vi "Continuous Input and Output.vi"() -> ()   [LabVIEW 2014]
doc: "This example demonstrates how to continuously acquire buffered voltage measurements using a DAQmx device.\n\nFor instructions on how to connect your signals to the DAQ device, refer to your device documentation."
uses:
  <vilib>/Utility/error.llb/DialogType.ctl
  <vilib>/DAQmx/read.llb/DAQmx Read (Analog 1D Wfm NChan NSamp).vi
  <vilib>/DAQmx/write.llb/DAQmx Write (Analog 1D DBL NChan 1Samp).vi
  <vilib>/DAQmx/create/channels.llb/DAQmx Create Channel (AI-Voltage-Basic).vi
  <vilib>/DAQmx/configure/timing.llb/DAQmx Timing (Sample Clock).vi
  <vilib>/DAQmx/create/channels.llb/DAQmx Create Channel (AO-Voltage-Basic).vi
  <vilib>/DAQmx/miscellaneous.llb/DAQmx Fill In Error Info.vi
  <vilib>/measure/madcrms.llb/Basic Averaged DC-RMS for 1 Chan.vi
  <vilib>/express/express analysis/Spectral/Block/exnSpectralBlock spectral measurements power poly.vi
  <vilib>/express/express analysis/Spectral/Block/exnSpectralBlock spectral measurements power WFM.vi
  <vilib>/express/express analysis/Spectral/XNode/ExpressSpectralMeasurementsBlockNode.xnode
  <resource>/objmgr/daqmx.rc
  <vilib>/measure/NI_MAPro.lvlib
panel:
  in  "Lower Cut-Off":dbl=100.0
  in  "Channel to Filter":i32
  out "Spectrum":cluster{"f0":dbl, "df":dbl, "magnitude":dbl[]}(graph)
  out "Filtered Data":waveform(dbl)(graph)
  in  "Physical Channel(s)":tag="Dev1/ao0"
  in  "Stop":bool
  out "Waveform Graph":waveform(dbl)[](graph)
  in  "Number of Samples":i32=100
  in  "Sample Rate":dbl=1000.0
  in  "Sample Clock Source":tag="OnboardClock"
  in  "Terminal Configuration":i32(ring)=-1 items=["default"=-1, "RSE"=10083, "NRSE"=10078, "Differential"=10106, "Pseudodifferential"=12529]
  in  "Max Voltage":dbl=5.0
  in  "Min Voltage":dbl
  in  "Physical Input Channel":tag="Dev1/ai0"
  out "Actual Sample Rate":dbl=1000.0 format="%0.2f"
  # "Channel Settings"
  # "Acquired Data"
  # "Filtered Data"
  # "Timing Settings"
  # "Spectrum"
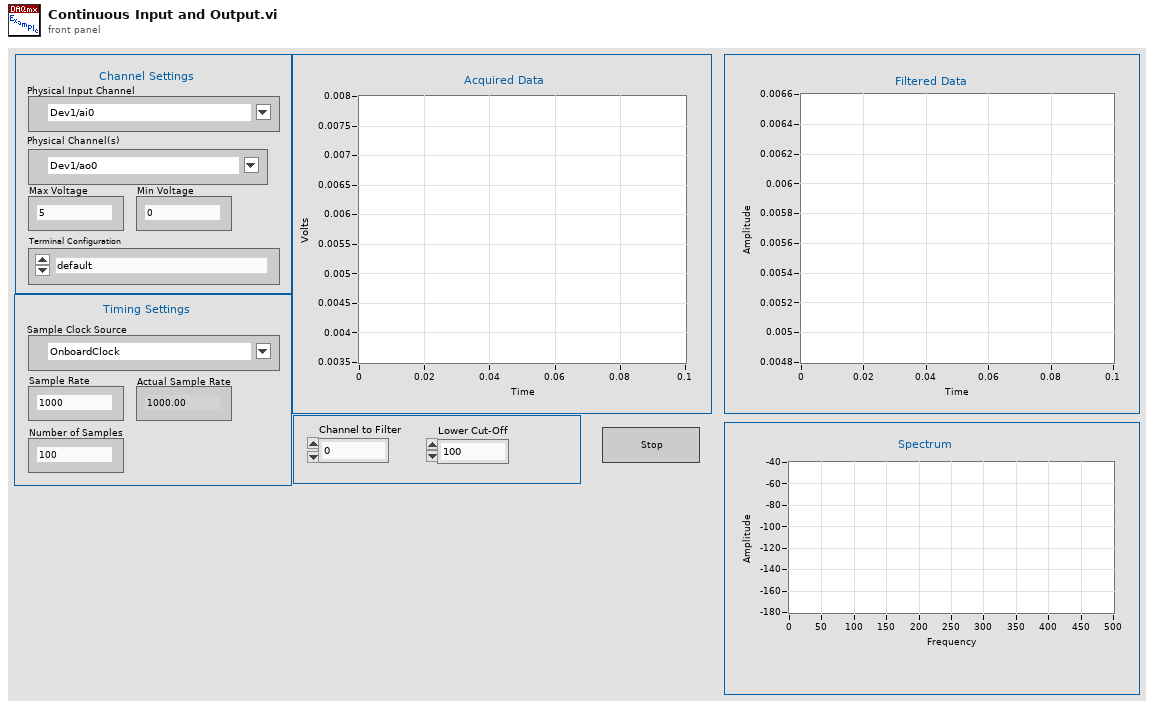
[diagram p1: front panel]
types:
  T1 = typedef "DialogType.ctl" = u16
  T2 = cluster{"averaging mode":u16, "weighting mode":u16, "number of averages":u32}
  T3 = cluster{"dB On (F)":bool, "unwrap phase (F)":bool, "convert to degree (F)":bool}
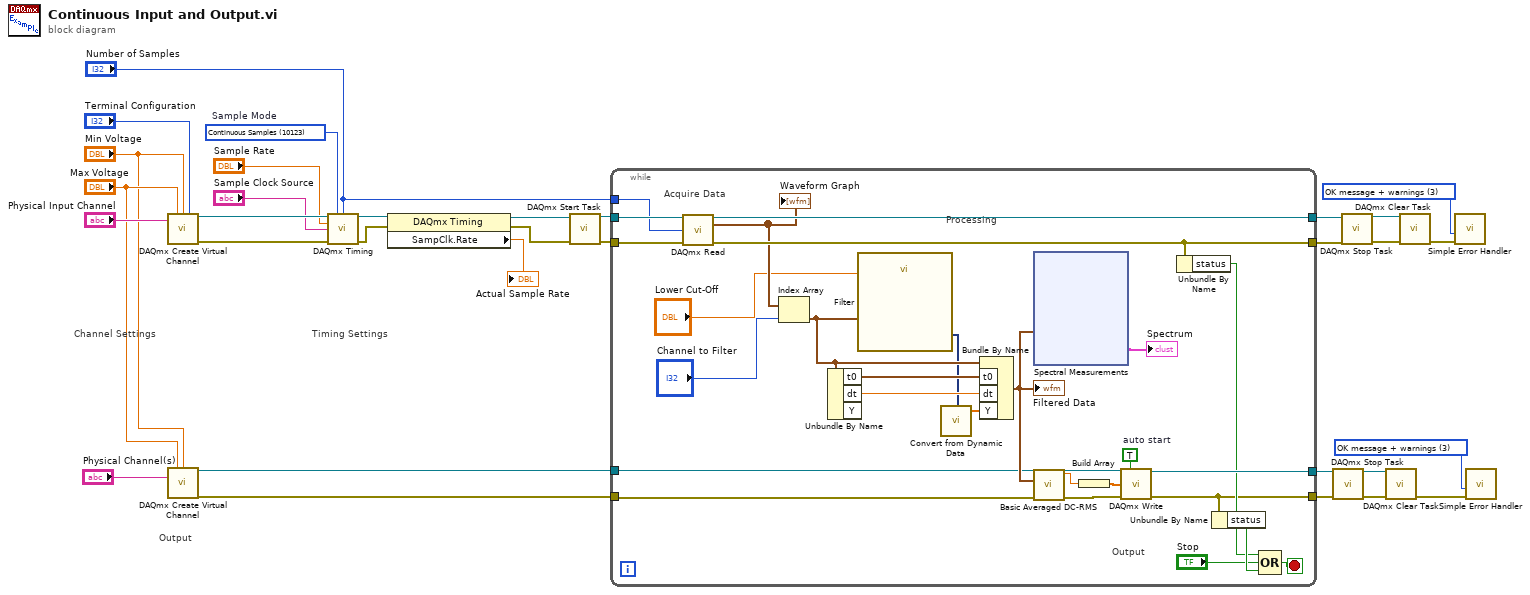
[diagram p0: block diagram]
diagram:
  w7 = T1 3 items=["no dialog", "OK message", "continue or stop message", "OK message + warnings", "continue/stop + warnings"] ("type of dialog (OK msg:1)")
  w17 = T1 3 items=["no dialog", "OK message", "continue or stop message", "OK message + warnings", "continue/stop + warnings"] ("type of dialog (OK msg:1)")
  w11 = 10123 items=["Finite Samples"=10178, "Continuous Samples"=10123, "Hardware Timed Single Point"=12522]  # Sample Mode
  # "Output"
  # "Timing Settings"
  # "Channel Settings"
  n1 = call-poly <vilib>:"DAQmx Create Virtual Channel.vi"("maximum value"="Max Voltage", "minimum value"="Min Voltage", "input terminal configuration"="Terminal Configuration", "physical channels"="Physical Input Channel") -> ("task out"=w29:refnum<k21>, "error out"=w30:errorcluster)  [unwired: 10 in]
  n2 = call-poly <vilib>:"DAQmx Create Virtual Channel.vi"("maximum value"="Max Voltage", "minimum value"="Min Voltage", "physical channels"="Physical Channel(s)") -> ("task out"=w2:refnum<k21>, "error out"=w1:errorcluster)  [unwired: 11 in]
  n3 = call-poly <vilib>:"DAQmx Timing.vi"("task/channels in"=w29, "sample mode"=w11, "samples per channel"="Number of Samples", "rate"="Sample Rate", "source"="Sample Clock Source", "error in"=w30) -> ("task out"=w32:refnum<k21>, "error out"=w31:errorcluster)  [unwired: 8 in]
  n4 = property class="DAQmx Timing"(reference=w32, error in=w31) -> (reference out=w4:refnum<k21>, error out=w3:errorcluster, "SampClk.Rate"=→"Actual Sample Rate":dbl)
  n5 = call <vilib>:"DAQmx Start Task.vi"("task/channels in"=w4, "error in"=w3) -> ("task out"=w28:refnum<k21>, "error out"=w27:errorcluster)  [unwired: 12 in]
  n6 = while {
    tunnel: w28 -> [w59]
    tunnel: w27 -> [w58]
    tunnel: [w57] -> w21
    tunnel: [w56] -> w20
    tunnel: "Number of Samples" -> [w55]
    tunnel: [w54] -> w6
    tunnel: [w39] -> w5
    tunnel: w2 -> [w34]
    tunnel: w1 -> [w33]
    stop <- w50 stop-if-true
    w38 = TRUE  # auto start
    # "Output"
    # "Processing"
    # "Acquire Data"
    n7 = call-poly <vilib>:"DAQmx Read.vi"("task/channels in"=w59, "number of samples per channel"=w55, "error in"=w58) -> ("task out"=w57:refnum<k21>, "data"=w49:waveform(dbl)[], "error out"=w56:errorcluster)  [unwired: 10 in]
    "Waveform Graph" <- w49
    n8 = Index Array(array=w49, index="Channel to Filter") -> (element=w47:waveform(dbl))
    n9 = Unbundle By Name(w47) -> ("t0"=w46:timestamp, "dt"=w45:dbl)  [unwired: 1 out]
    n10 = call "Filter"("Lower Cut-Off"="Lower Cut-Off", "Signal"=w47) -> ("Filtered Signal"=w40:dynamicdata)  [unwired: 8 in, 1 out]
    n11 = call "Convert from Dynamic Data"("Dynamic Data Type"=w40) -> ("Array"=w44:dbl[])  [unwired: 3 in]
    n12 = Bundle By Name(cluster=w47, "t0"=w46, "dt"=w45, "Y"=w44) -> (w42:waveform(dbl))
    "Filtered Data" <- w42
    n13 = xnode "Spectral Measurements"("Signals"=w42) -> ("Power Spectrum"=→"Spectrum":cluster{"f0":dbl, "df":dbl, "magnitude":dbl[]})  [unwired: 1 in, 1 out]
    n14 = call-poly <vilib>:"Basic Averaged DC-RMS.vi"("error in (no error)"=w33, "signal in"=w42) -> ("error out"=w37:errorcluster, "DC value"=w36:dbl)  [unwired: 6 in, 2 out]
    n15 = Build Array(w36) -> (w35:dbl[])
    n16 = call-poly <vilib>:"DAQmx Write.vi"("task/channels in"=w34, "auto start"=w38, "data"=w35, "error in"=w37) -> ("task out"=w54:refnum<k21>, "error out"=w39:errorcluster)  [unwired: 9 in, 1 out]
    n17 = Unbundle By Name(w56) -> ("status"=w51:bool)
    n18 = Unbundle By Name(w39) -> ("status"=w53:bool)
    n19 = Compound Arithmetic op=OR(w51, "Stop", w53) -> (w50:bool)
  }
  n20 = call <vilib>:"DAQmx Stop Task.vi"("task/channels in"=w6, "error in"=w5) -> ("task out"=w9:refnum<k21>, "error out"=w8:errorcluster)  [unwired: 12 in]
  n21 = call <vilib>:"DAQmx Stop Task.vi"("task/channels in"=w21, "error in"=w20) -> ("task out"=w18:refnum<k21>, "error out"=w19:errorcluster)  [unwired: 12 in]
  n22 = call <vilib>:"DAQmx Clear Task.vi"("task in"=w9, "error in"=w8) -> ("error out"=w10:errorcluster)  [unwired: 13 in]
  n23 = call <vilib>:"DAQmx Clear Task.vi"("task in"=w18, "error in"=w19) -> ("error out"=w26:errorcluster)  [unwired: 13 in]
  n24 = call <vilib>:"Simple Error Handler.vi"("type of dialog (OK msg:1)"=w17, "error in (no error)"=w26) -> ()  [unwired: 3 in, 5 out]
  n25 = call <vilib>:"Simple Error Handler.vi"("type of dialog (OK msg:1)"=w7, "error in (no error)"=w10) -> ()  [unwired: 3 in, 5 out]
